vi "Prueba de labiew.vi"(0 "Offset":dbl(knob) scale=0.0..10.0, 2 "Reset Signal":bool, 5 "Frecuencia":dbl(knob)=10.1 caption="Frequency" scale=0.0..500.0, 7 "Amplitud (V)":dbl(knob)=1.0 caption="Amplitude" scale=0.0..10.0, 9 "Fase":dbl(knob) caption="Phase" scale=-90.0..90.0, 11 "error in (no error)":errorcluster) -> (4 "Sine":dynamicdata(graph), 15 "error out":errorcluster)   [LabVIEW 2020]
doc: "Simulates a sine wave, square wave, triangle wave, sawtooth wave, or noise signal.\n--------------------\n\nThis Express VI is configured as follows:\n\nSignal Type: Sine\nFrequency: 10,1 Hz\nAmplitude: 1\nPhase: 0\nOffset: 0\nSampling Rate: 1000 Hz\nNumber of Samples: 100 (Automatic)\nTiming: Run as fast as possible\nTimestamps: Relative"
panel:
  in  "Ruido":bool=TRUE
  in  "Noise Ring":u16(ring) items=["Uniform White Noise", "Gaussian White Noise", "Periodic Random Noise", "Gamma Noise", "Poisson Noise", "Binomial Noise", "Bernoulli Noise", "MLS Sequence "]
  in  "Generate":u16(ring) items=["Sine", "Square", "Triangle", "Sawtooth", "DC"]
  in  "stop":bool
  in  "Trials":i32=1
  in  "Seed Number":dbl=-1.0
  in  "Amplitud del ruido(V)":dbl(knob)=0.6 caption="Noise amplitude" step=0.1 scale=0.0..10.0
  in  "Ciclo de Trabajo (%)":dbl(knob)=50.0 caption="Duty Cycle (%)" scale=0.0..100.0
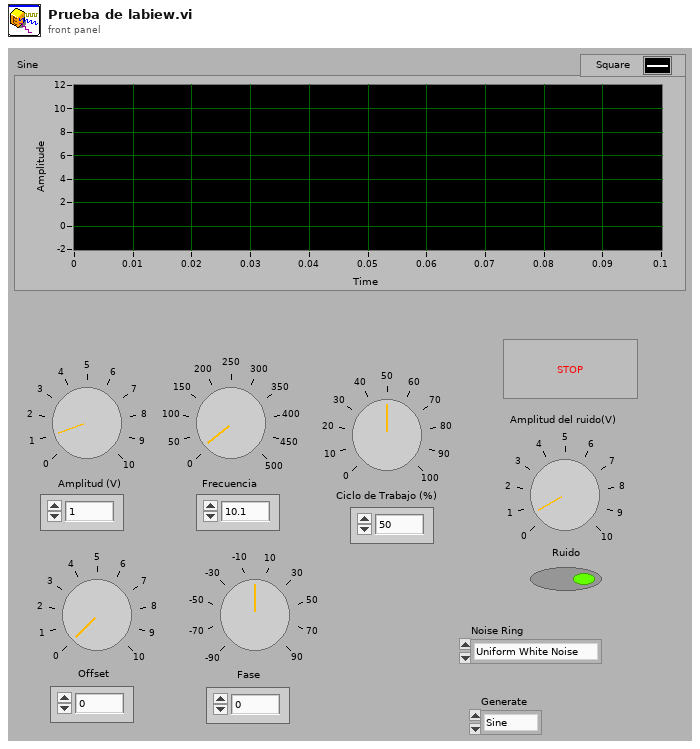
[diagram p1: front panel]
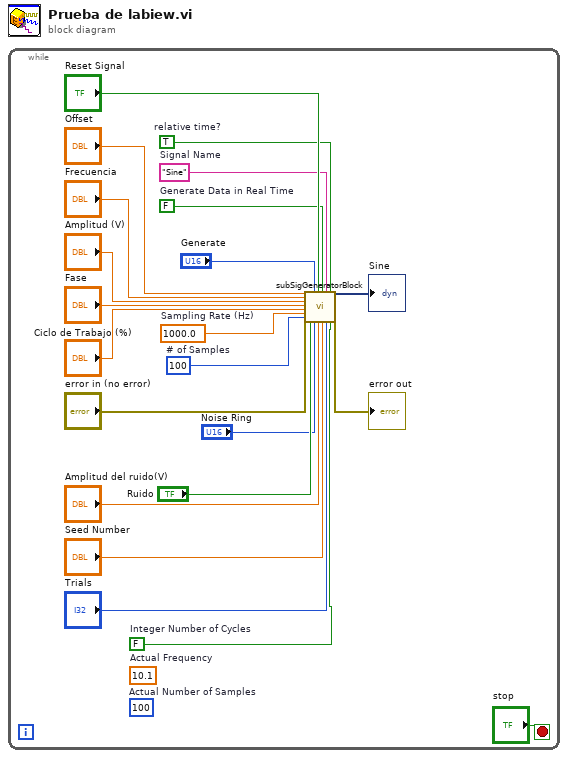
[diagram p0: block diagram]
diagram:
  n1 = while {
    stop <- "stop" stop-if-true
    (unwired) 10.1  # Actual Frequency
    (unwired) 100  # Actual Number of Samples
    w2 = FALSE  # Integer Number of Cycles
    w10 = TRUE  # relative time?
    w11 = "Sine"  # Signal Name
    w12 = FALSE  # Generate Data in Real Time
    w16 = 100  # # of Samples
    w18 = 1000.0  # Sampling Rate (Hz)
    n2 = call <vilib>:"subSigGeneratorBlock.vi"("Offset"="Offset", "Frequency"="Frecuencia", "Amplitude"="Amplitud (V)", "Phase"="Fase", "Duty Cycle (%)"="Ciclo de Trabajo (%)", "Sampling Rate (Hz)"=w18, "# of Samples"=w16, "error in (no error)"="error in (no error)", "Noise"="Ruido", "Generate"="Generate", "Noise Ring"="Noise Ring", "Reset Signal"="Reset Signal", "Noise Amplitude"="Amplitud del ruido(V)", "Generate Data in Real Time"=w12, "Seed Number"="Seed Number", "Signal Name"=w11, "trials"="Trials", "relative time?"=w10, "Integer Number of Cycles"=w2) -> ("Signal"=→"Sine":dynamicdata, "error out"=→"error out":errorcluster)  [unwired: 7 in]
  }
